vi "TestStand Version.vi"(8 "error in (no error)":errorcluster, 11 "Engine in":refnum<class "Engine.lvclass">) -> (0 "error out":errorcluster, 2 "VersionString":string, 3 "Engine out":refnum<class "Engine.lvclass">)   [LabVIEW 2020, in "TSnax.lvlib" / "Engine.lvclass"]
uses:
  Engine.lvclass
  Engine.lvclass/Engine.ctl
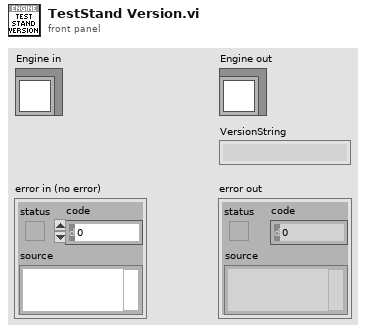
[diagram p1: front panel]
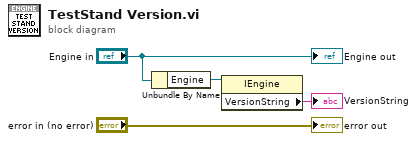
[diagram p0: block diagram]
diagram:
  n1 = Unbundle By Name("Engine in") -> ("Engine"=w2:refnum<k7>)
  n2 = property class="IEngine"(reference=w2) -> ("VersionString"=→"VersionString":string)  [unwired: 1 in, 2 out]
  "error out" <- "error in (no error)"
  "Engine out" <- "Engine in"
